vi "Random number 0-10.vi"() -> ()   [LabVIEW 2018]
panel:
  out "Meter":dbl(knob) scale=0.0..10.0
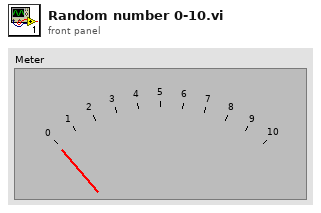
[diagram p1: front panel]
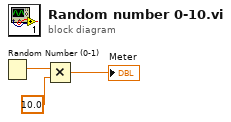
[diagram p0: block diagram]
diagram:
  n1 = Random Number (0-1)() -> (number: 0 to 1=w3:dbl)
  n2 = Multiply(x=w3, y=10.0) -> (x*y=→"Meter":dbl)
